vi "ExAdvAppCamera.vi"() -> ()   [LabVIEW 2010]
uses:
  Open-Close/CamHandle.vi
  GlobalInitializeFlag.vi
  GlobalFramesToStr.vi
  GlobalTimingMode.vi
  GlobalAcquireFocusFlag.vi
  GlobalExposure.vi
  GlobalUserBin.vi
  GlobalBin2x.vi
  GlobalFullBin.vi
  GlobalCCDMaxDim.vi
  GlobalFlipFlag.vi
  GlobalReverseFlag.vi
  GlobalIBackImgHndl.vi
  GlobalIFlatImgHndl.vi
panel:
  out "Camera Opened":bool
  in  "Exit program":bool
  out "error out":errorcluster
  in  "error in (no error)":errorcluster
  in  "Tab Control":T1(tab)
  in  "Focus/Acquire Mode":u32=1 min=1 max=5 step=1
  in  "Number of Frames to store":u32=1 min=1 step=1
  in  "Intensifier":bool
  in  "Readout Port":i32=-1 min=-1 step=1
  in  "ADC Offset 2":i32=-1 min=-1 step=1
  in  "ADC Gain 2":i32=-1 min=-1 step=1
  in  "ADC speed":i32=-2 min=-3 step=1
  in  "Trigger Edge":u32(ring)=1 items=["N/A", "Positive (leading) edge", "Negative (falling) edge"]
  in  "Timing Mode":u32(ring)=1 items=["N/A", "Free Run/Timed", "Trigger First (PM only)", "Ext Sync/Strobed ", "Variable Exp (PM only)", "Flash Mode (PM only)"]
  out "Pixel Time":i32
  out "Bit Depth":i32
  out "ReadOut port":i32
  out "ADC Offset":i32
  out "ADC Gain":i32
  out "ADC Speed":i32
  in  "Set Experiment \nParameters, Initialize \nCamera/Controller":bool
  out "temperature":dbl format="%.2f"
  out "Temperature Read":dbl(slide) scale=-120.0..20.0
  in  "Temperature":dbl format="%.2f"
  in  "Exposure":dbl format="%.2f"
  out "Controller Initialized":bool
  out "Total":u32
  out "Y dim":u32
  out "X dim":u32
  in  "Y Bin":u32=1 min=1 step=1
  in  "Y End":u32=100 min=1 step=1
  in  "Y Start":u32=1 min=1 step=1
  in  "X Bin":u32=1 min=1 step=1
  in  "X End":u32=100 min=1 step=1
  in  "X Start":u32=1 min=1 step=1
  out "Bin 2":bool
  out "User":bool
  out "Full":bool
  in  "Binned by 2 Button":bool
  in  "User Defined Button":bool
  in  "Full CCD Button":bool
  out "Flip\nActive":bool
  in  "Flip flag Button":bool
  out "Reverse\nActive":bool
  in  "Image Reverse Button":bool
  out "Flat Field\nActive":bool
  out "Background \nActive":bool
  in  "Frame number to read":u32=1 min=1 step=1
  in  "Flat Button":bool
  in  "Back Button":bool
  in  "Full File Name":path
  in  "FileType":u32=67371008
  in  "SITKFULLDISPLAYLib.SITKFullDisplay":refnum<k7>(container)
  out "Reverse\nactive":bool
  out "Flip\nactive":bool
  out "Flat Field\nactive":bool
  out "background\nactive":bool
  in  "Reverse\nbutton":bool
  in  "Flip\nbutton":bool
  in  "Flat Field\nbutton":bool
  in  "Background\nbutton":bool
  in  "stop 2":bool
  in  "Start":bool
  out "Camera initialized":bool
  out "Collecting Data":bool
  in  "SITKFULLDISPLAYLib.SITKFullDisplay":refnum<k7>(container)
  in  "Full File Name\nfor Acqure":path
  in  "OK Button":bool
  out "camera initialized":bool
  # "Note: In order for any parameters to change and be downloaded the initialize button must be hit."
  # "The following are read \nfrom camera after setting\nvalues to left.\n-1 value means it isn't \nsupported by camera."
  # "For Slowest ADC speed set this to -3\nFor Fastest ADC speed set this to -2\nTo use current ADC speed don't  hook up or use -1\notherwise put speed in as kHz"
  # "To use current gain don't hook up or set to -1"
  # "To use current gain don't hook up or set to -1"
  # "To use current gain don't hook up or set to -1"
  # "NOTE: if background subtraction and/or flat field are being used and the ROi\nis changed, there are checks in this example for size compatability."
  # "Pixels coming back\nfrom Camera"
  # "File Types:\nSPE = 67371008\nTIF   = 67174400\nPMI  = 67436544"
  # "Browse match pattern is set to *.spe.  Modify this if different file type is needed."
  # "Instructions:\nMake sure camera/controller has been initialized, led should be on.\nPress start button, display should appear.\nWhen done press stop button, display should disappear.\nLive Operations buttons only work while collecting data, not before.  To setup before goto Live operations tab."
  # "Live Oerations, will only work while collecting data."
  # "Instructions:\nMake sure the camera/controller has been initialized, (the light should be on).\nMake sure to put in a file name with path to save data.\nPress Start button and display will pop up and data will be saved in file."
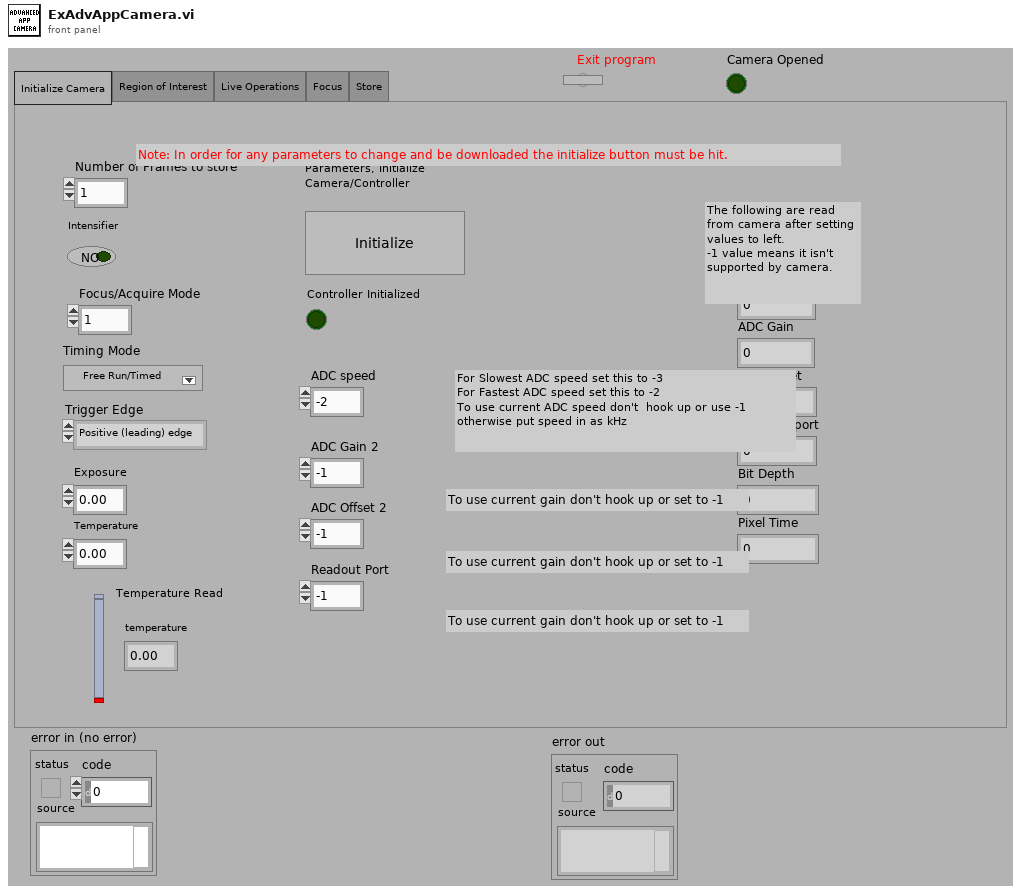
[diagram p1: front panel]
types:
  T1 = enum32{"Initialize Camera", "Region of Interest", "Live Operations", "Focus", "Store"}
  T2 = cluster{"X Start":u32, "X End":u32, "X Bin":u32, "Y Start":u32, "Y End":u32, "Y Bin":u32}
  T3 = cluster{i32, "CCD Max X":u32, i32, i32, "CCD Max Y":u32, i32}
  T4 = cluster{"Camera Handle":u32, "Pulser Handle":u32, "File Handle":u32, "Display Handle":u32, "Image Handle":u32}
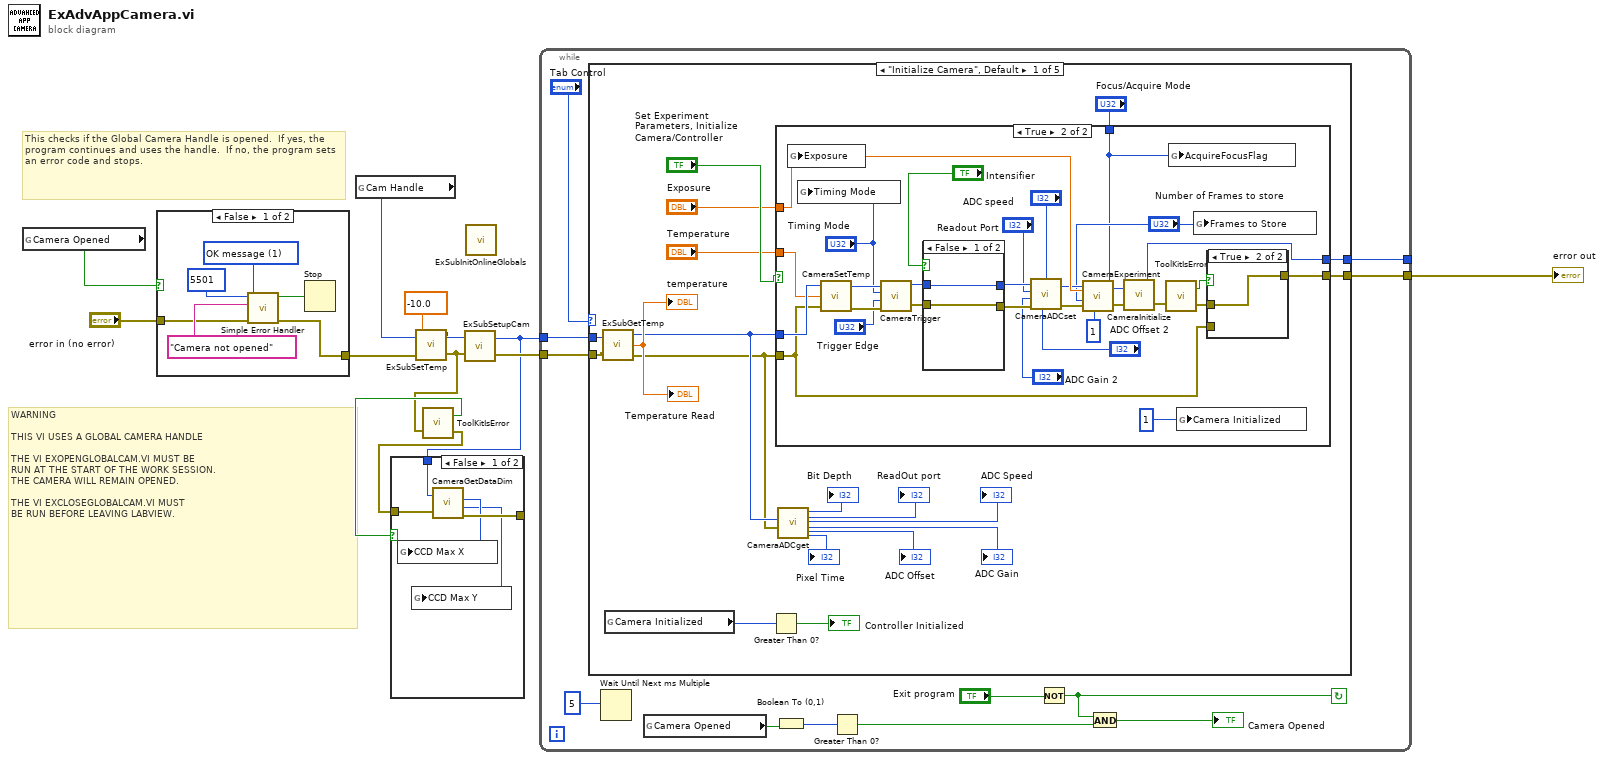
[diagram p0: block diagram]
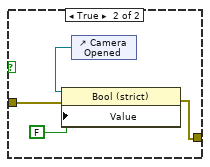
[diagram p3: hidden frame]
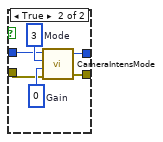
[diagram p6: hidden frame]
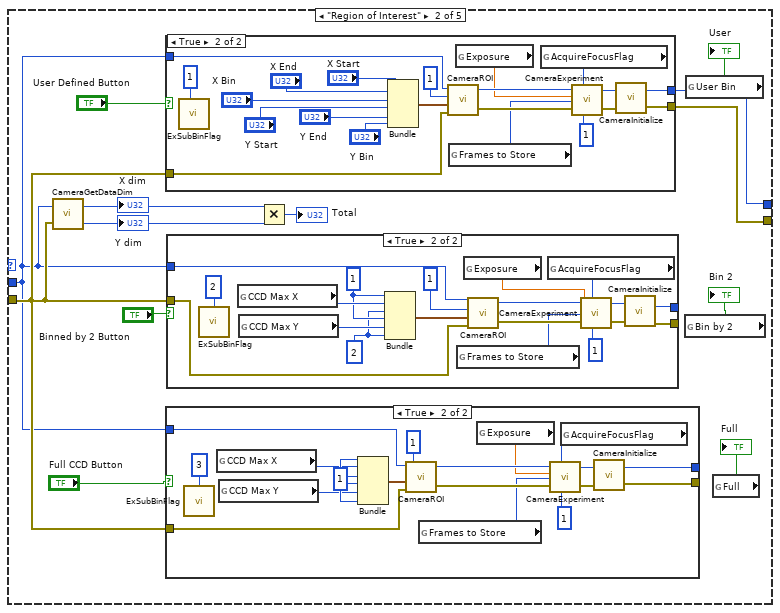
[diagram p7: hidden frame]
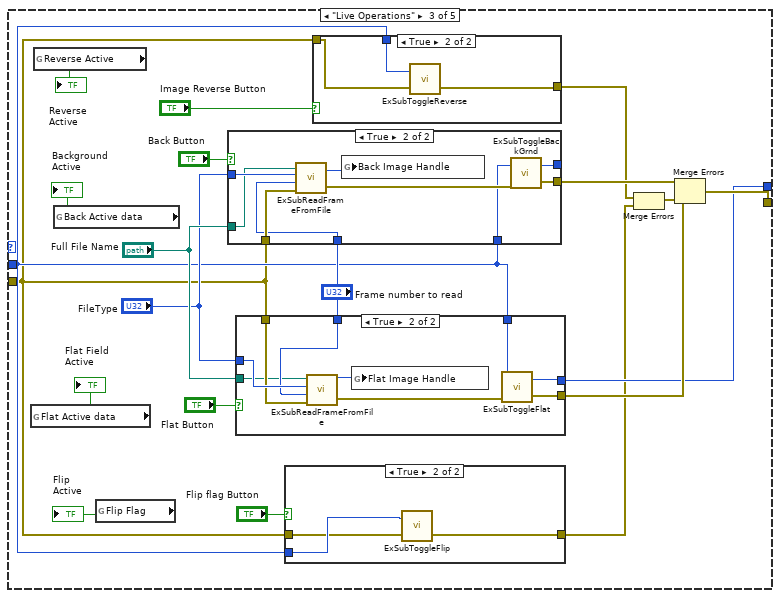
[diagram p11: hidden frame]
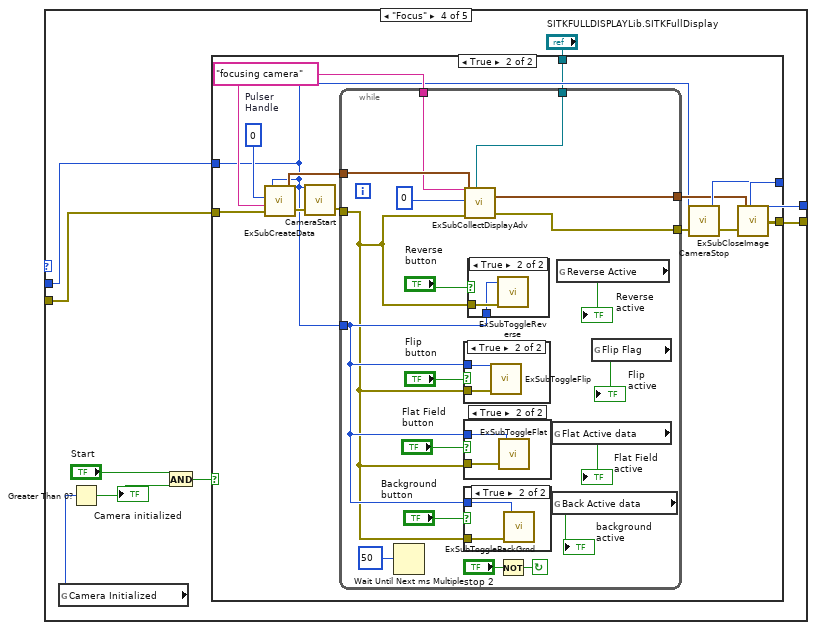
[diagram p16: hidden frame]
diagram:
  # "WARNING\n\nTHIS VI USES A GLOBAL CAMERA HANDLE\n\nTHE VI EXOPENGLOBALCAM.VI MUST BE\nRUN AT THE START OF THE WORK SESSION.\nTHE CAMERA WILL REMAIN OPENED.\n\nTHE VI EXCLOSEGLOBALCAM.VI MUST\nBE RUN BEFORE LEAVING LABVIEW."
  # "This checks if the Global Camera Handle is opened.  If yes, the program continues and uses the handle.  If no, the program sets\nan error code and stops."
  n1 = global read "CamHandle.vi" "Camera Opened"() -> (w7:bool)
  n2 = case shown="False" w7 {
    tunnel: "error in (no error)" -> [w14 w20]
    tunnel: [w13 w19] -> w8
    frame False {
      w18 = u16 1 items=["no dialog", "OK message", "continue or stop message"] ("type of dialog (OK msg:1)")
      n3 = call <vilib>:"Simple Error Handler.vi"("error code (no error:0)"=5501, "error source (\" \")"="Camera not opened", "type of dialog (OK msg:1)"=w18, "error in (no error)"=w14) -> ("error?"=w16:bool, "error out"=w13:errorcluster)  [unwired: 1 in, 3 out]
      n4 = Stop(stop? (T)=w16) -> ()
    }
    frame True {
      n5 = control-ref of="Camera Opened"() -> (w21:refnum<vi>)
      n6 = property class="Bool (strict)"(reference=w21, error in=w20, "Value"=FALSE) -> (error out=w19:errorcluster)  [unwired: 1 out]
    }
  }
  n7 = global read "CamHandle.vi" "Cam Handle"() -> (w9:u32)
  n8 = call "ExSubSetTemp.vi"("error in (no error)"=w8, "Temperature"=-10.0, "CameraHandle"=w9) -> ("error out"=w1:errorcluster, "Camera Handle"=w11:u32)
  n9 = call <userlib>:"ToolKitIsError.vi"("error in"=w1) -> ("error out"=w3:errorcluster, "Error Flag"=w4:bool)  [unwired: 1 in]
  n10 = call "ExSubSetupCam.vi"("error in (no error)"=w1, "Camera Handle"=w11) -> ("error out"=w5:errorcluster, "Camera Handle"=w2:u32)
  n11 = case shown="False" w4 {
    tunnel: w3 -> [w26 w28]
    tunnel: [w27 w28] -> _
    tunnel: w2 -> [w23 _]
    frame False {
      n12 = call <userlib>:"CameraGetDataDim.vi"("Camera Handle"=w23, "error in"=w26) -> ("Xdim"=w25:u32, "Ydim"=w24:u32, "error out"=w27:errorcluster)  [unwired: 1 out]
      n13 = global write "GlobalCCDMaxDim.vi" "CCD Max X"(w25) -> ()
      n14 = global write "GlobalCCDMaxDim.vi" "CCD Max Y"(w24) -> ()
    }
    frame True {
    }
  }
  n15 = call "ExSubInitOnlineGlobals.vi"() -> ()  [unwired: 1 in]
  n16 = while {
    tunnel: w2 -> [w40]
    tunnel: w5 -> [w37]
    tunnel: [w36] -> _
    tunnel: [w35] -> w6
    stop <- w34 continue-if-true
    n17 = case shown="\"Initialize Camera\", Default" "Tab Control" {
      tunnel: w40 -> [w59 w107 w183 w231 w284]
      tunnel: w37 -> [w51 w108 w182 w230 w283]
      tunnel: [w43 w106 w190 w233 w281] -> w36
      tunnel: [w42 w105 w191 w232 w282] -> w35
      frame "Initialize Camera", Default {
        n18 = call "ExSubGetTemp.vi"("Camera Handle"=w59, "error in (no error)"=w51) -> ("Camera Handle"=w50:u32, "Temperature Real"=→"temperature" →"Temperature Read":dbl, "error out"=w49:errorcluster)
        n19 = global read "GlobalInitializeFlag.vi" "Camera Initialized"() -> (w54:u32)
        n20 = Greater Than 0?(x=w54) -> (x > 0?=→"Controller Initialized":bool)
        n21 = case shown="True" "Set Experiment \nParameters, Initialize \nCamera/Controller" {
          tunnel: "Exposure" -> [_ w80]
          tunnel: "Temperature" -> [_ w89]
          tunnel: w49 -> [w60 w64]
          tunnel: w50 -> [w61 w90]
          tunnel: [w60 w67] -> w42
          tunnel: [w61 w65] -> w43
          tunnel: "Focus/Acquire Mode" -> [_ w62]
          frame False {
          }
          frame True {
            n22 = global write "GlobalExposure.vi" "Exposure"(w80) -> ()
            n23 = global write "GlobalTimingMode.vi" "Timing Mode"("Timing Mode") -> ()
            n24 = call <userlib>:"CameraSetTemp.vi"("error in (no error)"=w64, "Temperature"=w89, "Camera Handle"=w90) -> ("error out"=w79:errorcluster, "Camera Handle"=w78:u32)
            n25 = call <userlib>:"CameraTrigger.vi"("error in"=w79, "Trigger Edge"="Trigger Edge", "Timing Mode"="Timing Mode", "Camera Handle"=w78) -> ("error out"=w75:errorcluster, "Camera Handle"=w76:u32)
            n26 = case shown="False" "Intensifier" {
              tunnel: [w95 w101] -> w86
              tunnel: [w94 w100] -> w87
              tunnel: w76 -> [w95 w97]
              tunnel: w75 -> [w94 w96]
              frame False {
              }
              frame True {
                w98 = u32 0  # Gain
                w99 = u32 3  # Mode
                n27 = call <userlib>:"CameraIntensMode.vi"("error in"=w96, "Intensifier Gain"=w98, "Mode"=w99, "Camera Handle"=w97) -> ("error out"=w100:errorcluster, "Camera Handle"=w101:u32)
              }
            }
            n28 = call <userlib>:"CameraADCset.vi"("ADC offset"="ADC Offset 2", "Read Out port"="Readout Port", "error in (no error)"=w87, "ADC Gain"="ADC Gain 2", "ADC Speed"="ADC speed", "Camera Handle"=w86) -> ("error out"=w73:errorcluster, "Camera Handle"=w72:u32)
            n29 = call <userlib>:"CameraExperiment.vi"("Number of Accumulations"=1, "Acquire / Focus Flag"=w62, "error in"=w73, "Number of Images"="Number of Frames to store", "Exposure (sec)"=w80, "Camera Handle"=w72) -> ("error out"=w71:errorcluster, "Camera Handle"=w70:u32)
            n30 = call <userlib>:"CameraInitialize.vi"("error in"=w71, "Camera Handle"=w70) -> ("error out"=w66:errorcluster, "Camera Handle"=w65:u32)
            n31 = call <userlib>:"ToolKitIsError.vi"("error in"=w66) -> ("error out"=w68:errorcluster, "Error Flag"=w69:bool)  [unwired: 1 in]
            n32 = global write "GlobalAcquireFocusFlag.vi" "AcquireFocusFlag"(w62) -> ()
            n33 = global write "GlobalInitializeFlag.vi" "Camera Initialized"(1) -> ()
            n34 = global write "GlobalFramesToStr.vi" "Frames to Store"("Number of Frames to store") -> ()
            n35 = case shown="True" w69 {
              tunnel: w68 -> [_ w93]
              tunnel: [w92 w93] -> w67
              tunnel: w64 -> [w92 _]
              frame False {
              }
              frame True {
              }
            }
          }
        }
        n36 = call <userlib>:"CameraADCget.vi"("Camera handle"=w50, "error in (no error)"=w49) -> ("Bit Depth"=→"Bit Depth":i32, "Pixel Time"=→"Pixel Time":i32, "Readout Port"=→"ReadOut port":i32, "ADC Offset"=→"ADC Offset":i32, "ADC Speed"=→"ADC Speed":i32, "ADC Gain"=→"ADC Gain":i32)  [unwired: 2 out]
      }
      frame "Region of Interest" {
        n37 = call <userlib>:"CameraGetDataDim.vi"("Camera Handle"=w107, "error in"=w108) -> ("Xdim"=w104:u32, "Ydim"=w103:u32)  [unwired: 2 out]
        "X dim" <- w104
        "Y dim" <- w103
        n38 = case shown="True" "User Defined Button" {
          tunnel: w107 -> [w157 w161]
          tunnel: [w157 w176] -> w106
          tunnel: w108 -> [w156 w160]
          tunnel: [w156 w173] -> w105
          frame False {
          }
          frame True {
            n39 = call "ExSubBinFlag.vi"("Binning \nUser = 1\nBin 2 = 2\nFull = 3"=1) -> ()
            n40 = Bundle("X Start"="X Start", "X End"="X End", "X Bin"="X Bin", "Y Start"="Y Start", "Y End"="Y End", "Y Bin"="Y Bin") -> (w162:T2)  [unwired: 1 in]
            n41 = call <userlib>:"CameraROI.vi"("error in"=w160, "ROI Params"=w162, "ROI Index"=1, "Camera Handle"=w161) -> ("error out"=w175:errorcluster, "Camera Handle"=w178:u32)
            n42 = global read "GlobalFramesToStr.vi" "Frames to Store"() -> (w170:u32)
            n43 = global read "GlobalExposure.vi" "Exposure"() -> (w171:dbl)
            n44 = global read "GlobalAcquireFocusFlag.vi" "AcquireFocusFlag"() -> (w169:u32)
            n45 = call <userlib>:"CameraExperiment.vi"("Number of Accumulations"=1, "Acquire / Focus Flag"=w169, "error in"=w175, "Number of Images"=w170, "Exposure (sec)"=w171, "Camera Handle"=w178) -> ("error out"=w174:errorcluster, "Camera Handle"=w177:u32)
            n46 = call <userlib>:"CameraInitialize.vi"("error in"=w174, "Camera Handle"=w177) -> ("error out"=w173:errorcluster, "Camera Handle"=w176:u32)
          }
        }
        n47 = case shown="True" "Full CCD Button" {
          tunnel: w107 -> [w116 w119]
          tunnel: [w116 w126] -> _
          tunnel: w108 -> [w115 w118]
          tunnel: [w115 w125] -> _
          frame False {
          }
          frame True {
            w124 = 1
            n48 = call "ExSubBinFlag.vi"("Binning \nUser = 1\nBin 2 = 2\nFull = 3"=3) -> ()
            n49 = global read "GlobalCCDMaxDim.vi" "CCD Max X"() -> (w123:u32)
            n50 = global read "GlobalCCDMaxDim.vi" "CCD Max Y"() -> (w122:u32)
            n51 = Bundle(w124, "CCD Max X"=w123, w124, w124, "CCD Max Y"=w122, w124) -> (w121:T3)  [unwired: 1 in]
            n52 = call <userlib>:"CameraROI.vi"("error in"=w118, "ROI Params"=w121, "ROI Index"=1, "Camera Handle"=w119) -> ("error out"=w132:errorcluster, "Camera Handle"=w134:u32)
            n53 = global read "GlobalFramesToStr.vi" "Frames to Store"() -> (w128:u32)
            n54 = global read "GlobalExposure.vi" "Exposure"() -> (w129:dbl)
            n55 = global read "GlobalAcquireFocusFlag.vi" "AcquireFocusFlag"() -> (w127:u32)
            n56 = call <userlib>:"CameraExperiment.vi"("Number of Accumulations"=1, "Acquire / Focus Flag"=w127, "error in"=w132, "Number of Images"=w128, "Exposure (sec)"=w129, "Camera Handle"=w134) -> ("error out"=w131:errorcluster, "Camera Handle"=w133:u32)
            n57 = call <userlib>:"CameraInitialize.vi"("error in"=w131, "Camera Handle"=w133) -> ("error out"=w125:errorcluster, "Camera Handle"=w126:u32)
          }
        }
        n58 = case shown="True" "Binned by 2 Button" {
          tunnel: w107 -> [w136 w141]
          tunnel: [w136 w147] -> _
          tunnel: w108 -> [w135 w142]
          tunnel: [w135 w146] -> _
          frame False {
          }
          frame True {
            w138 = 2
            w139 = 1
            n59 = call "ExSubBinFlag.vi"("Binning \nUser = 1\nBin 2 = 2\nFull = 3"=2) -> ()
            n60 = global read "GlobalCCDMaxDim.vi" "CCD Max X"() -> (w145:u32)
            n61 = global read "GlobalCCDMaxDim.vi" "CCD Max Y"() -> (w144:u32)
            n62 = Bundle(w139, "CCD Max X"=w145, w138, w139, "CCD Max Y"=w144, w138) -> (w143:T3)  [unwired: 1 in]
            n63 = global read "GlobalFramesToStr.vi" "Frames to Store"() -> (w149:u32)
            n64 = global read "GlobalExposure.vi" "Exposure"() -> (w150:dbl)
            n65 = call <userlib>:"CameraROI.vi"("error in"=w142, "ROI Params"=w143, "ROI Index"=1, "Camera Handle"=w141) -> ("error out"=w153:errorcluster, "Camera Handle"=w155:u32)
            n66 = global read "GlobalAcquireFocusFlag.vi" "AcquireFocusFlag"() -> (w148:u32)
            n67 = call <userlib>:"CameraExperiment.vi"("Number of Accumulations"=1, "Acquire / Focus Flag"=w148, "error in"=w153, "Number of Images"=w149, "Exposure (sec)"=w150, "Camera Handle"=w155) -> ("error out"=w152:errorcluster, "Camera Handle"=w154:u32)
            n68 = call <userlib>:"CameraInitialize.vi"("error in"=w152, "Camera Handle"=w154) -> ("error out"=w146:errorcluster, "Camera Handle"=w147:u32)
          }
        }
        n69 = Multiply(x=w104, y=w103) -> (x*y=→"Total":u32)
        n70 = global read "GlobalBin2x.vi" "Bin by 2"() -> (→"Bin 2":bool)
        n71 = global read "GlobalUserBin.vi" "User Bin"() -> (→"User":bool)
        n72 = global read "GlobalFullBin.vi" "Full"() -> (→"Full":bool)
      }
      frame "Live Operations" {
        n73 = global read "GlobalIFlatImgHndl.vi" "Flat Active data"() -> (→"Flat Field\nActive":bool)
        n74 = global read "GlobalReverseFlag.vi" "Reverse Active"() -> (→"Reverse\nActive":bool)
        n75 = global read "GlobalIBackImgHndl.vi" "Back Active data"() -> (→"Background \nActive":bool)
        n76 = global read "GlobalFlipFlag.vi" "Flip Flag"() -> (→"Flip\nActive":bool)
        n77 = case shown="True" "Back Button" {
          tunnel: "Full File Name" -> [_ w226]
          tunnel: "FileType" -> [_ w227]
          tunnel: w182 -> [w219 w228]
          tunnel: [w219 w222] -> w193
          tunnel: "Frame number to read" -> [_ w225]
          tunnel: w183 -> [w218 w221]
          tunnel: [w218 w220] -> _
          frame False {
          }
          frame True {
            n78 = call "ExSubReadFrameFromFile.vi"("error in (no error)"=w228, "Frame to extract"=w225, "File type"=w227, "path to file to open"=w226) -> ("error out"=w223:errorcluster, "Image Handle"=w224:u32)
            n79 = global write "GlobalIBackImgHndl.vi" "Back Image Handle"(w224) -> ()
            n80 = call "ExSubToggleBackGrnd.vi"("error in (no error)"=w223, "Camera Handle"=w221) -> ("error out"=w222:errorcluster, "Camera Handle"=w220:u32)
          }
        }
        n81 = case shown="True" "Flat Button" {
          tunnel: "Full File Name" -> [_ w214]
          tunnel: "FileType" -> [_ w217]
          tunnel: w182 -> [w208 w215]
          tunnel: [w208 w210] -> w192
          tunnel: "Frame number to read" -> [_ w216]
          tunnel: w183 -> [w207 w212]
          tunnel: [w207 w211] -> w190
          frame False {
          }
          frame True {
            n82 = call "ExSubReadFrameFromFile.vi"("error in (no error)"=w215, "Frame to extract"=w216, "File type"=w217, "path to file to open"=w214) -> ("error out"=w209:errorcluster, "Image Handle"=w213:u32)
            n83 = global write "GlobalIFlatImgHndl.vi" "Flat Image Handle"(w213) -> ()
            n84 = call "ExSubToggleFlat.vi"("error in (no error)"=w209, "Camera Handle"=w212) -> ("error out"=w210:errorcluster, "Camera Handle"=w211:u32)
          }
        }
        n85 = case shown="True" "Flip flag Button" {
          tunnel: w183 -> [_ w206]
          tunnel: w182 -> [w203 w205]
          tunnel: [w203 w204] -> w181
          frame False {
          }
          frame True {
            n86 = call "ExSubToggleFlip.vi"("error in (no error)"=w205, "Camera Handle"=w206) -> ("error out"=w204:errorcluster)  [unwired: 1 out]
          }
        }
        n87 = case shown="True" "Image Reverse Button" {
          tunnel: w183 -> [_ w201]
          tunnel: w182 -> [w199 w202]
          tunnel: [w199 w200] -> w180
          frame False {
          }
          frame True {
            n88 = call "ExSubToggleReverse.vi"("error in (no error)"=w202, "Camera Handle"=w201) -> ("error out"=w200:errorcluster)  [unwired: 1 out]
          }
        }
        n89 = Merge Errors(w180, w181) -> (w179:errorcluster)
        n90 = Merge Errors(w193, w192, w179) -> (w191:errorcluster)
      }
      frame "Focus" {
        n91 = global read "GlobalInitializeFlag.vi" "Camera Initialized"() -> (w235:u32)
        n92 = Greater Than 0?(x=w235) -> (x > 0?=w234:bool)
        "Camera initialized" <- w234
        n93 = And(x="Start", y=w234) -> (x .and. y?=w237:bool)
        n94 = case shown="True" w237 {
          tunnel: w230 -> [w238 w248]
          tunnel: w231 -> [w239 w241]
          tunnel: [w239 w245] -> w233
          tunnel: [w238 w244] -> w232
          tunnel: "SITKFULLDISPLAYLib.SITKFullDisplay" -> [_ w240]
          frame False {
          }
          frame True {
            w242 = "focusing camera"
            w249 = u32 0  # Pulser  Handle
            n95 = call "ExSubCreateData.vi"("error in (no error)"=w248, "File and Display Name"=w242, "Pulser Handle"=w249, "Camera Handle"=w241) -> ("error out"=w250:errorcluster, "Handles Out"=w252:T4)
            n96 = call <userlib>:"CameraStart.vi"("error in"=w250, "Camera Handle"=w241) -> ("error out"=w251:errorcluster)  [unwired: 1 out]
            n97 = while {
              tunnel: w252 -> [w270]
              tunnel: w251 -> [w259]
              tunnel: [w269] -> w247
              tunnel: [w253] -> w243
              tunnel: w242 -> [w265]
              tunnel: w241 -> [w260]
              tunnel: w240 -> [w254]
              stop <- w267 continue-if-true
              n98 = Wait Until Next ms Multiple(millisecond multiple=u32 50) -> ()  [unwired: 1 out]
              n99 = case shown="True" "Flip\nbutton" {
                tunnel: w260 -> [_ w276]
                tunnel: w259 -> [_ w277]
                frame False {
                }
                frame True {
                  n100 = call "ExSubToggleFlip.vi"("error in (no error)"=w277, "Camera Handle"=w276) -> ()  [unwired: 2 out]
                }
              }
              n101 = case shown="True" "Flat Field\nbutton" {
                tunnel: w260 -> [_ w274]
                tunnel: w259 -> [_ w275]
                frame False {
                }
                frame True {
                  n102 = call "ExSubToggleFlat.vi"("error in (no error)"=w275, "Camera Handle"=w274) -> ()  [unwired: 2 out]
                }
              }
              n103 = case shown="True" "Background\nbutton" {
                tunnel: w260 -> [_ w273]
                tunnel: w259 -> [_ w272]
                frame False {
                }
                frame True {
                  n104 = call "ExSubToggleBackGrnd.vi"("error in (no error)"=w272, "Camera Handle"=w273) -> ()  [unwired: 2 out]
                }
              }
              n105 = call "ExSubCollectDisplayAdv.vi"("Handle Cluster"=w270, "Display Title"=w265, "Store flag"=0, "error in (no error)"=w259, "advanced display handle"=w254) -> ("Handle Cluster Out"=w253:T4, "error out"=w269:errorcluster)  [unwired: 1 out]
              n106 = case shown="True" "Reverse\nbutton" {
                tunnel: w259 -> [_ w279]
                tunnel: w260 -> [_ w278]
                frame False {
                }
                frame True {
                  n107 = call "ExSubToggleReverse.vi"("error in (no error)"=w279, "Camera Handle"=w278) -> ()  [unwired: 2 out]
                }
              }
              n108 = Not(x="stop 2") -> (.not. x?=w267:bool)
              n109 = global read "GlobalIFlatImgHndl.vi" "Flat Active data"() -> (→"Flat Field\nactive":bool)
              n110 = global read "GlobalIBackImgHndl.vi" "Back Active data"() -> (→"background\nactive":bool)
              n111 = global read "GlobalReverseFlag.vi" "Reverse Active"() -> (→"Reverse\nactive":bool)
              n112 = global read "GlobalFlipFlag.vi" "Flip Flag"() -> (→"Flip\nactive":bool)
            }
            n113 = call <userlib>:"CameraStop.vi"("error in"=w247, "Camera Handle"=w241) -> ("error out"=w246:errorcluster, "Camera Handle"=w245:u32)
            n114 = call "ExSubCloseImage.vi"("error in (no error)"=w246, "Handles In"=w243) -> ("error out"=w244:errorcluster)
          }
        }
      }
      frame "Store" {
        n115 = global read "GlobalInitializeFlag.vi" "Camera Initialized"() -> (w286:u32)
        n116 = Greater Than 0?(x=w286) -> (x > 0?=w285:bool)
        "camera initialized" <- w285
        n117 = And(x="OK Button", y=w285) -> (x .and. y?=w288:bool)
        n118 = case shown="True" w288 {
          tunnel: w284 -> [w290 w303]
          tunnel: w283 -> [w289 w293]
          tunnel: [w289 w296] -> w282
          tunnel: [w290 w303] -> w281
          frame False {
          }
          frame True {
            w306 = u32 0  # Pulser Handle
            n119 = property on="Collecting Data" class="Bool (strict)"(error in=w293, "Value"=TRUE) -> (error out=w292:errorcluster)  [unwired: 1 in, 1 out]
            n120 = Path To String(path="Full File Name\nfor Acqure") -> (string=w304:string)
            n121 = call "ExSubCreateFile.vi"("error in (no error)"=w292, "File and Display Name"=w304, "Pulser Handle"=w306, "Camera Handle"=w303) -> ("error out"=w307:errorcluster, "Handles Out"=w299:T4)
            n122 = call <userlib>:"CameraStart.vi"("error in"=w307, "Camera Handle"=w303) -> ("error out"=w300:errorcluster, "Camera Handle"=w297:u32)
            n123 = global read "GlobalFramesToStr.vi" "Frames to Store"() -> (w298:u32)
            n124 = call "ExSubNframeAdv.vi"("error in (no error)"=w300, "Display handle"="SITKFULLDISPLAYLib.SITKFullDisplay", "Number of Images"=w298, "Handle Cluster"=w299) -> ("error out"=w294:errorcluster, "Handle Cluster"=w302:T4)
            n125 = call <userlib>:"CameraStop.vi"("error in"=w294, "Camera Handle"=w297) -> ("error out"=w301:errorcluster)  [unwired: 1 out]
            n126 = call "ExSubCloseFileImage.vi"("error in (no error)"=w301, "Handles In"=w302) -> ("error out"=w296:errorcluster)
          }
        }
        "Collecting Data" <- FALSE
      }
    }
    n127 = Wait Until Next ms Multiple(millisecond multiple=5) -> ()  [unwired: 1 out]
    n128 = global read "CamHandle.vi" "Camera Opened"() -> (w31:bool)
    n129 = Boolean To (0,1)(Boolean=w31) -> (0, 1=w30:i16)
    n130 = Greater Than 0?(x=w30) -> (x > 0?=w29:bool)
    n131 = Not(x="Exit program") -> (.not. x?=w34:bool)
    n132 = And(x=w34, y=w29) -> (x .and. y?=→"Camera Opened":bool)
  }
  "error out" <- w6
